vi "Get Adjustment.vi"(8 "error in (no error)":errorcluster) -> (0 "error out":errorcluster, 3 "Adjustment Value (0-1)":dbl)   [LabVIEW 2015]
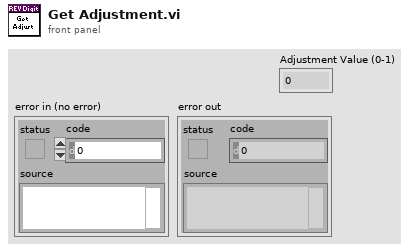
[diagram p1: front panel]
types:
  T1 = typedef "WPI_AnalogChannelDevRef.ctl" = cluster{"DevStatus":errorcluster, "Analog Channel":T2}
  T2 = typedef "FPGA_AIChannel.ctl" = enum8{"AI 0", "AI 1", "AI 2", "AI 3", "AI MXP 0", "AI MXP 1", "AI MXP 2", "AI MXP 3", "Invalid"}
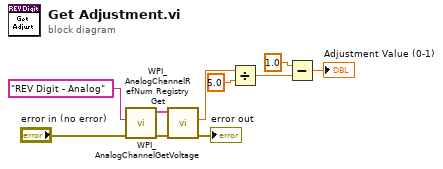
[diagram p0: block diagram]
diagram:
  n1 = call <vilib>:"WPI_AnalogChannelRefNum Registry Get.vi"("error in (no error)"="error in (no error)", "refnum name"="REV Digit - Analog") -> ("error out"=w9:errorcluster, "AIDeviceRef"=w10:T1)  [unwired: 8 in]
  n2 = call <vilib>:"WPI_AnalogChannelGetVoltage.vi"("error in (no error)"=w9, "AIDeviceRef"=w10) -> ("error out"=→"error out":errorcluster, "Voltage"=w4:dbl)  [unwired: 7 in, 1 out]
  n3 = Divide(x=w4, y=5.0) -> (x/y=w3:dbl)
  n4 = Subtract(x=1.0, y=w3) -> (x-y=→"Adjustment Value (0-1)":dbl)
